vi "Get_Continuous_Angle.vi"(5 "Device Number":T1) -> (3 "Continuous Angle":T2)   [LabVIEW 2017]
uses:
  Kauai Labs/labviewae/_TypeDefs/FRIC_navX_DeviceNumbersTypeDef.ctl
panel:
  in  "Zero":bool
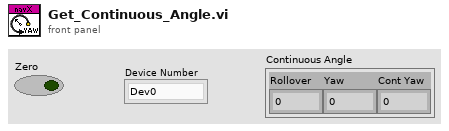
[diagram p1: front panel]
types:
  T1 = typedef "FRIC_navX_DeviceNumbersTypeDef.ctl" = enum16{"Dev0", "Dev1", "Dev2", "Dev3", "Dev4", "Dev5", "Dev6", "Dev7", "Dev8", "Dev9", "Dev10"}
  T2 = cluster{"Rollover":dbl, "Yaw":dbl, "Cont Yaw":dbl}
  T3 = cluster{"Yaw":dbl, "Roll":dbl, "Pitch":dbl, "Heading":dbl, "Fused Heading":dbl}
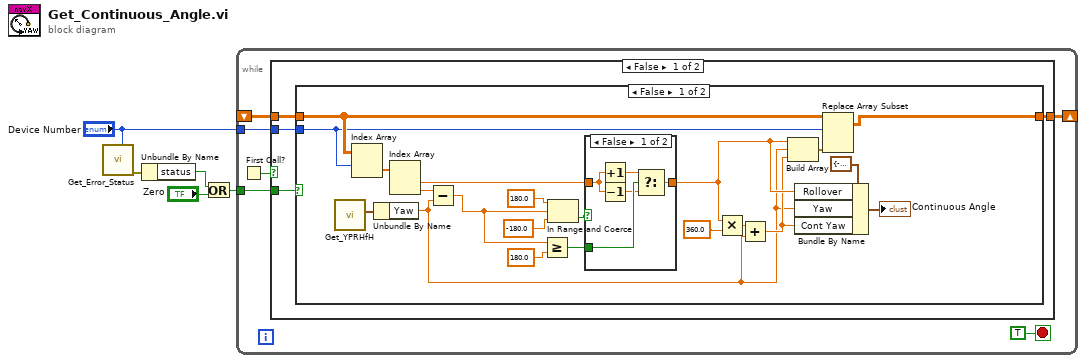
[diagram p0: block diagram]
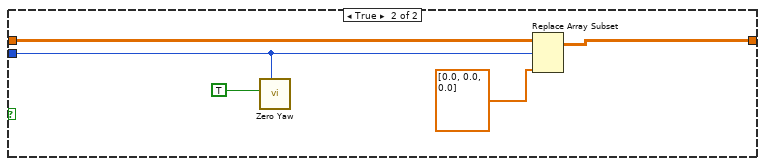
[diagram p3: hidden frame]
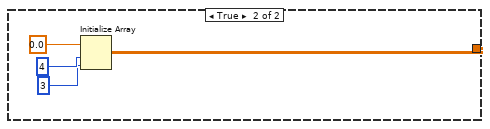
[diagram p4: hidden frame]
diagram:
  n1 = call <vilib>:"Get_Error_Status.vi"("Device Number"="Device Number") -> ("error out"=w3:errorcluster)  [unwired: 10 in]
  n2 = Unbundle By Name(w3) -> ("status"=w1:bool)
  n3 = Or(x=w1, y="Zero") -> (x .or. y?=w2:bool)
  n4 = while {
    shift-right: [w9] -> _
    shift-left: _ -> [w10]
    tunnel: "Device Number" -> [w8]
    tunnel: w2 -> [w6]
    stop <- TRUE stop-if-true
    n5 = First Call?() -> (First Call?: T/F=w7:bool)
    n6 = case shown="False" w7 {
      tunnel: w10 -> [w15 _]
      tunnel: [w14 w51] -> w9
      tunnel: w8 -> [w13 _]
      tunnel: w6 -> [w12 _]
      frame False {
        n7 = case shown="False" w12 {
          tunnel: w15 -> [w36 w47]
          tunnel: [w35 w46] -> w14
          tunnel: w13 -> [w34 w44]
          frame False {
            n8 = call "Get_YPRHfH.vi"() -> ("YRPHfH"=w29:T3)  [unwired: 11 in]
            n9 = Index Array(array=w36, index (row)=w34) -> (element=w33:dbl[])  [unwired: 1 in]
            n10 = Unbundle By Name(w29) -> ("Yaw"=w16:dbl)
            n11 = Index Array(array=w33) -> (element #1=w32:dbl, element #2=w31:dbl)  [unwired: 2 in]
            n12 = Subtract(x=w31, y=w16) -> (x-y=w20:dbl)
            n13 = Greater Or Equal?(x=w20, y=180.0) -> (x >= y?=w22:bool)
            n14 = In Range and Coerce(upper limit=180.0, x=w20, lower limit=-180.0) -> (In Range?=w19:bool)  [unwired: 1 out]
            n15 = case shown="False" w19 {
              tunnel: w32 -> [w41 w42]
              tunnel: [w40 w42] -> w24
              tunnel: w22 -> [w39 _]
              frame False {
                n16 = Increment(x=w41) -> (x+1=w38:dbl)
                n17 = Decrement(x=w41) -> (x-1=w37:dbl)
                n18 = Select(t=w38, s=w39, f=w37) -> (s? t:f=w40:dbl)
              }
              frame True {
              }
            }
            n19 = Multiply(x=w24, y=360.0) -> (x*y=w28:dbl)
            n20 = Add(x=w28, y=w16) -> (x+y=w21:dbl)
            n21 = Build Array(w24, w16, w21) -> (w30:dbl[])
            n22 = Bundle By Name(cluster=T2 {"Rollover"=-0.34, "Yaw"=0.2, "Cont Yaw"=0.2} ("YRPHfH"), "Rollover"=w24, "Yaw"=w16, "Cont Yaw"=w21) -> (→"Continuous Angle":T2)
            n23 = Replace Array Subset(array=w36, new element=w30, index (row)=w34) -> (w35:dbl[][])  [unwired: 1 in]
          }
          frame True {
            n24 = call <vilib>:"Zero Yaw.vi"("Device Number"=w44, "Zero"=TRUE) -> ()  [unwired: 10 in]
            n25 = Replace Array Subset(array=w47, new element=dbl[] [0.0, 0.0, 0.0] ("new element/subarray"), index (row)=w44) -> (w46:dbl[][])  [unwired: 1 in]
          }
        }
      }
      frame True {
        n26 = Initialize Array(0.0, 4, 3 ("dimension size")) -> (w51:dbl[][])
      }
    }
  }
